vi "example_02_convert.vi"() -> ()   [LabVIEW 2015, in "lv-unit-conversion.lvlib"] (continued)
Kingdom 2240 lbf."}, {"symbol"="tonf[US]", "name"="US ton-force", "dimension"="LM/T2", "is_si_unit"=TRUE, "category"="atom", "base_unit"="N", "conversion_reference"="NIST-SI", "is_exact"=TRUE, "a"=0.0, "b"=8896.443230521, "c"=1.0, "d"=0.0, "underlying_def"="2000 lbf", "description"="2000 lbf"}, {"symbol"="J.m/m2", "name"="joule metre per square metre", "dimension"="LM/T2", "is_si_unit"=TRUE, "category"="derived", "base_unit"="", "conversion_reference"="", "is_exact"=FALSE, "a"=0.0, "b"=0.0, "c"=0.0, "d"=0.0, "underlying_def"="N", "description"=""}, {"symbol"="J/m", "name"="joule per metre", "dimension"="LM/T2", "is_si_unit"=TRUE, "category"="derived", "base_unit"="", "conversion_reference"="", "is_exact"=FALSE, "a"=0.0, "b"=0.0, "c"=0.0, "d"=0.0, "underlying_def"="N", "description"=""}, {"symbol"="N.m/m", "name"="newton metre per metre", "dimension"="LM/T2", "is_si_unit"=TRUE, "category"="derived", "base_unit"="", "conversion_reference"="", "is_exact"=FALSE, "a"=0.0, "b"=0.0, "c"=0.0, "d"=0.0, "underlying_def"="N", "description"=""}, {"symbol"="kcal[th].m/cm2", "name"="thousand calorie metre per square centimetre", "dimension"="LM/T2", "is_si_unit"=TRUE, "category"="derived", "base_unit"="J.m/m2", "conversion_reference"="DERIVED", "is_exact"=TRUE, "a"=0.0, "b"=41840000.0, "c"=1.0, "d"=0.0, "underlying_def"="", "description"=""}, {"symbol"="MJ/m", "name"="megajoule per metre", "dimension"="LM/T2", "is_si_unit"=TRUE, "category"="derived", "base_unit"="J/m", "conversion_reference"="DERIVED", "is_exact"=TRUE, "a"=0.0, "b"=1000000.0, "c"=1.0, "d"=0.0, "underlying_def"="", "description"=""}, {"symbol"="10 kN", "name"="ten kilonewton", "dimension"="LM/T2", "is_si_unit"=TRUE, "category"="derived", "base_unit"="N", "conversion_reference"="DERIVED", "is_exact"=TRUE, "a"=0.0, "b"=10000.0, "c"=1.0, "d"=0.0, "underlying_def"="", "description"=""}, {"symbol"="kgf.m/m", "name"="thousand gram-force metre per metre", "dimension"="LM/T2", "is_si_unit"=TRUE, "category"="derived", "base_unit"="N.m/m", "conversion_reference"="DERIVED", "is_exact"=TRUE, "a"=0.0, "b"=9.80665, "c"=1.0, "d"=0.0, "underlying_def"="", "description"=""}, {"symbol"="lbf.ft/in", "name"="foot pound-force per inch", "dimension"="LM/T2", "is_si_unit"=TRUE, "category"="derived", "base_unit"="N.m/m", "conversion_reference"="DERIVED", "is_exact"=TRUE, "a"=0.0, "b"=53.378659383126, "c"=1.0, "d"=0.0, "underlying_def"="", "description"="Equivalent to \"12 lbf\"."}, {"symbol"="lbf.in/in", "name"="pound-force inch per inch", "dimension"="LM/T2", "is_si_unit"=TRUE, "category"="derived", "base_unit"="N.m/m", "conversion_reference"="DERIVED", "is_exact"=TRUE, "a"=0.0, "b"=4.4482216152605, "c"=1.0, "d"=0.0, "underlying_def"="", "description"=""}, {"symbol"="tonf[US].mi/ft", "name"="US ton-force mile per foot", "dimension"="LM/T2", "is_si_unit"=TRUE, "category"="derived", "base_unit"="N.m/m", "conversion_reference"="DERIVED", "is_exact"=TRUE, "a"=0.0, "b"=46973220.25715088, "c"=1.0, "d"=0.0, "underlying_def"="", "description"="Equivalent to \"5280 tonf[US]\"."}, {"symbol"="cN", "name"="centinewton", "dimension"="LM/T2", "is_si_unit"=TRUE, "category"="prefixed", "base_unit"="N", "conversion_reference"="DERIVED", "is_exact"=TRUE, "a"=0.0, "b"=0.01, "c"=1.0, "d"=0.0, "underlying_def"="", "description"=""}, {"symbol"="daN", "name"="dekanewton", "dimension"="LM/T2", "is_si_unit"=TRUE, "category"="prefixed", "base_unit"="N", "conversion_reference"="DERIVED", "is_exact"=TRUE, "a"=0.0, "b"=10.0, "c"=1.0, "d"=0.0, "underlying_def"="", "description"=""}, {"symbol"="dN", "name"="decinewton", "dimension"="LM/T2", "is_si_unit"=TRUE, "category"="prefixed", "base_unit"="N", "conversion_reference"="DERIVED", "is_exact"=TRUE, "a"=0.0, "b"=0.1, "c"=1.0, "d"=0.0, "underlying_def"="", "description"=""}, {"symbol"="EN", "name"="exanewton", "dimension"="LM/T2", "is_si_unit"=TRUE, "category"="prefixed", "base_unit"="N", "conversion_reference"="DERIVED", "is_exact"=TRUE, "a"=0.0, "b"=1e+18, "c"=1.0, "d"=0.0, "underlying_def"="", "description"=""}, {"symbol"="fN", "name"="femtonewton", "dimension"="LM/T2", "is_si_unit"=TRUE, "category"="prefixed", "base_unit"="N", "conversion_reference"="DERIVED", "is_exact"=TRUE, "a"=0.0, "b"=1e-15, "c"=1.0, "d"=0.0, "underlying_def"="", "description"=""}, {"symbol"="GN", "name"="giganewton", "dimension"="LM/T2", "is_si_unit"=TRUE, "category"="prefixed", "base_unit"="N", "conversion_reference"="DERIVED", "is_exact"=TRUE, "a"=0.0, "b"=1000000000.0, "c"=1.0, "d"=0.0, "underlying_def"="", "description"=""}, {"symbol"="hN", "name"="hectonewton", "dimension"="LM/T2", "is_si_unit"=TRUE, "category"="prefixed", "base_unit"="N", "conversion_reference"="DERIVED", "is_exact"=TRUE, "a"=0.0, "b"=100.0, "c"=1.0, "d"=0.0, "underlying_def"="", "description"=""}, {"symbol"="kdyne", "name"="kilodyne", "dimension"="LM/T2", "is_si_unit"=TRUE, "category"="prefixed", "base_unit"="N", "conversion_reference"="DERIVED", "is_exact"=TRUE, "a"=0.0, "b"=0.01, "c"=1.0, "d"=0.0, "underlying_def"="", "description"=""}, {"symbol"="kgf", "name"="thousand gram-force", "dimension"="LM/T2", "is_si_unit"=TRUE, "category"="prefixed", "base_unit"="N", "conversion_reference"="DERIVED", "is_exact"=TRUE, "a"=0.0, "b"=9.80665, "c"=1.0, "d"=0.0, "underlying_def"="", "description"=""}, {"symbol"="klbf", "name"="thousand pound-force", "dimension"="LM/T2", "is_si_unit"=TRUE, "category"="prefixed", "base_unit"="N", "conversion_reference"="DERIVED", "is_exact"=TRUE, "a"=0.0, "b"=4448.2216152605, "c"=1.0, "d"=0.0, "underlying_def"="", "description"=""}, {"symbol"="kN", "name"="kilonewton", "dimension"="LM/T2", "is_si_unit"=TRUE, "category"="prefixed", "base_unit"="N", "conversion_reference"="DERIVED", "is_exact"=TRUE, "a"=0.0, "b"=1000.0, "c"=1.0, "d"=0.0, "underlying_def"="", "description"=""}, {"symbol"="Mgf", "name"="million gram-force", "dimension"="LM/T2", "is_si_unit"=TRUE, "category"="prefixed", "base_unit"="N", "conversion_reference"="DERIVED", "is_exact"=TRUE, "a"=0.0, "b"=9806.65, "c"=1.0, "d"=0.0, "underlying_def"="", "description"=""}, {"symbol"="mN", "name"="millinewton", "dimension"="LM/T2", "is_si_unit"=TRUE, "category"="prefixed", "base_unit"="N", "conversion_reference"="DERIVED", "is_exact"=TRUE, "a"=0.0, "b"=0.001, "c"=1.0, "d"=0.0, "underlying_def"="", "description"=""}, {"symbol"="MN", "name"="meganewton", "dimension"="LM/T2", "is_si_unit"=TRUE, "category"="prefixed", "base_unit"="N", "conversion_reference"="DERIVED", "is_exact"=TRUE, "a"=0.0, "b"=1000000.0, "c"=1.0, "d"=0.0, "underlying_def"="", "description"=""}, {"symbol"="nN", "name"="nanonewton", "dimension"="LM/T2", "is_si_unit"=TRUE, "category"="prefixed", "base_unit"="N", "conversion_reference"="DERIVED", "is_exact"=TRUE, "a"=0.0, "b"=1e-09, "c"=1.0, "d"=0.0, "underlying_def"="", "description"=""}, {"symbol"="pN", "name"="piconewton", "dimension"="LM/T2", "is_si_unit"=TRUE, "category"="prefixed", "base_unit"="N", "conversion_reference"="DERIVED", "is_exact"=TRUE, "a"=0.0, "b"=1e-12, "c"=1.0, "d"=0.0, "underlying_def"="", "description"=""}, {"symbol"="TN", "name"="teranewton", "dimension"="LM/T2", "is_si_unit"=TRUE, "category"="prefixed", "base_unit"="N", "conversion_reference"="DERIVED", "is_exact"=TRUE, "a"=0.0, "b"=1000000000000.0, "c"=1.0, "d"=0.0, "underlying_def"="", "description"=""}, {"symbol"="uN", "name"="micronewton", "dimension"="LM/T2", "is_si_unit"=TRUE, "category"="prefixed", "base_unit"="N", "conversion_reference"="DERIVED", "is_exact"=TRUE, "a"=0.0, "b"=1e-06, "c"=1.0, "d"=0.0, "underlying_def"="", "description"=""}, {"symbol"="1/bar", "name"="per bar", "dimension"="LT2/M", "is_si_unit"=TRUE, "category"="derived", "base_unit"="1/Pa", "conversion_reference"="DERIVED", "is_exact"=TRUE, "a"=0.0, "b"=1e-05, "c"=1.0, "d"=0.0, "underlying_def"="", "description"=""}, {"symbol"="1/kPa", "name"="per kilopascal", "dimension"="LT2/M", "is_si_unit"=TRUE, "category"="derived", "base_unit"="1/Pa", "conversion_reference"="DERIVED", "is_exact"=TRUE, "a"=0.0, "b"=0.001, "c"=1.0, "d"=0.0, "underlying_def"="", "description"=""}, {"symbol"="1/pPa", "name"="per picopascal", "dimension"="LT2/M", "is_si_unit"=TRUE, "category"="derived", "base_unit"="1/Pa", "conversion_reference"="DERIVED", "is_exact"=TRUE, "a"=0.0, "b"=1000000000000.0, "c"=1.0, "d"=0.0, "underlying_def"="", "description"=""}, {"symbol"="1/psi", "name"="per psi", "dimension"="LT2/M", "is_si_unit"=TRUE, "category"="derived", "base_unit"="1/Pa", "conversion_reference"="DERIVED", "is_exact"=TRUE, "a"=0.0, "b"=0.00064516, "c"=4.4482216152605, "d"=0.0, "underlying_def"="", "description"=""}, {"symbol"="1/upsi", "name"="per millionth of psi", "dimension"="LT2/M", "is_si_unit"=TRUE, "category"="derived", "base_unit"="1/Pa", "conversion_reference"="DERIVED", "is_exact"=TRUE, "a"=0.0, "b"=645.16, "c"=4.4482216152605, "d"=0.0, "underlying_def"="", "description"=""}, {"symbol"="1/Pa", "name"="per pascal", "dimension"="LT2/M", "is_si_unit"=TRUE, "category"="derived", "base_unit"="", "conversion_reference"="", "is_exact"=FALSE, "a"=0.0, "b"=0.0, "c"=0.0, "d"=0.0, "underlying_def"="", "description"=""}, {"symbol"="m3/J", "name"="cubic metre per joule", "dimension"="LT2/M", "is_si_unit"=TRUE, "category"="derived", "base_unit"="", "conversion_reference"="", "is_exact"=FALSE, "a"=0.0, "b"=0.0, "c"=0.0, "d"=0.0, "underlying_def"="1/Pa", "description"=""}, {"symbol"="dm3/(kW.h)", "name"="cubic decimetre per kilowatt hour", "dimension"="LT2/M", "is_si_unit"=TRUE, "category"="derived", "base_unit"="m3/J", "conversion_reference"="DERIVED", "is_exact"=TRUE, "a"=0.0, "b"=0.001, "c"=3600000.0, "d"=0.0, "underlying_def"="", "description"=""}, {"symbol"="dm3/MJ", "name"="cubic decimetre per megajoule", "dimension"="LT2/M", "is_si_unit"=TRUE, "category"="derived", "base_unit"="m3/J", "conversion_reference"="DERIVED", "is_exact"=TRUE, "a"=0.0, "b"=1e-09, "c"=1.0, "d"=0.0, "underlying_def"="", "description"=""}, {"symbol"="m3/(kW.h)", "name"="cubic metre per kilowatt hour", "dimension"="LT2/M", "is_si_unit"=TRUE, "category"="derived", "base_unit"="m3/J", "conversion_reference"="DERIVED", "is_exact"=TRUE, "a"=0.0, "b"=1.0, "c"=3600000.0, "d"=0.0, "underlying_def"="", "description"=""}, {"symbol"="mm3/J", "name"="cubic millimetre per joule", "dimension"="LT2/M", "is_si_unit"=TRUE, "category"="derived", "base_unit"="m3/J", "conversion_reference"="DERIVED", "is_exact"=TRUE, "a"=0.0, "b"=1e-09, "c"=1.0, "d"=0.0, "underlying_def"="", "description"=""}, {"symbol"="pt[UK]/(hp.h)", "name"="UK pint per horsepower hour", "dimension"="LT2/M", "is_si_unit"=TRUE, "category"="derived", "base_unit"="m3/J", "conversion_reference"="DERIVED", "is_exact"=TRUE, "a"=0.0, "b"=0.00056826125, "c"=2684519.537696173, "d"=0.0, "underlying_def"="", "description"=""}, {"symbol"="ct", "name"="carat", "dimension"="M", "is_si_unit"=TRUE, "category"="atom", "base_unit"="kg", "conversion_reference"="NIST-SI", "is_exact"=TRUE, "a"=0.0, "b"=0.0002, "c"=1.0, "d"=0.0, "underlying_def"="200 mg", "description"="200 milligrams (exactly), from NIST-44."}, {"symbol"="cwt[UK]", "name"="UK hundredweight", "dimension"="M", "is_si_unit"=TRUE, "category"="atom", "base_unit"="kg", "conversion_reference"="UK-1995", "is_exact"=TRUE, "a"=0.0, "b"=50.80234544, "c"=1.0, "d"=0.0, "underlying_def"="112 lbm", "description"="United Kingdom 112 pound-mass Gross or long hundredweight. From NIST-44."}, {"symbol"="cwt[US]", "name"="US hundredweight", "dimension"="M", "is_si_unit"=TRUE, "category"="atom", "base_unit"="kg", "conversion_reference"="NIST-44", "is_exact"=TRUE, "a"=0.0, "b"=45.359237, "c"=1.0, "d"=0.0, "underlying_def"="100 lbm", "description"="100 lbm. Net or short hundredweight. From NIST-44."}, {"symbol"="g", "name"="gram", "dimension"="M", "is_si_unit"=TRUE, "category"="atom-base", "base_unit"="kg", "conversion_reference"="NIST-SI", "is_exact"=TRUE, "a"=0.0, "b"=0.001, "c"=1.0, "d"=0.0, "underlying_def"="1/1000 kg", "description"="One thousandth of a kilogram."}, {"symbol"="grain", "name"="grain", "dimension"="M", "is_si_unit"=TRUE, "category"="atom", "base_unit"="kg", "conversion_reference"="NIST-44", "is_exact"=TRUE, "a"=0.0, "b"=6.479891e-05, "c"=1.0, "d"=0.0, "underlying_def"="", "description"="The \"grain\" is the same in avoirdupois, troy, and apothecaries units of mass."}, {"symbol"="lbm", "name"="pound-mass", "dimension"="M", "is_si_unit"=TRUE, "category"="atom", "base_unit"="kg", "conversion_reference"="NIST-SI", "is_exact"=TRUE, "a"=0.0, "b"=0.45359237, "c"=1.0, "d"=0.0, "underlying_def"="", "description"="International avoirdupois pound."}, {"symbol"="ozm", "name"="ounce-mass", "dimension"="M", "is_si_unit"=TRUE, "category"="atom", "base_unit"="kg", "conversion_reference"="NIST-44", "is_exact"=TRUE, "a"=0.0, "b"=0.45359237, "c"=16.0, "d"=0.0, "underlying_def"="1/16 lbm", "description"="One sixteenth of an International avoirdupois pound (lbm)."}, {"symbol"="ozm[troy]", "name"="troy ounce-mass", "dimension"="M", "is_si_unit"=TRUE, "category"="atom", "base_unit"="kg", "conversion_reference"="NIST-44", "is_exact"=TRUE, "a"=0.0, "b"=0.0311034768, "c"=1.0, "d"=0.0, "underlying_def"="480 grain", "description"="Apothecaries or Troy ounce"}, {"symbol"="sack[94lbm]", "name"="94 pound-mass sack", "dimension"="M", "is_si_unit"=TRUE, "category"="atom", "base_unit"="kg", "conversion_reference"="DEFINITION", "is_exact"=TRUE, "a"=0.0, "b"=42.63768278, "c"=1.0, "d"=0.0, "underlying_def"="94 lbm", "description"="A sack with a nominal weight of 94 pound-mass. \n\t\t\t\tWhile the conversion of 94 lbm is exact, the weight of the sack is not exactly 94 lbm.\n\t\t\t"}, {"symbol"="t", "name"="tonne", "dimension"="M", "is_si_unit"=TRUE, "category"="atom-allowed", "base_unit"="kg", "conversion_reference"="NIST-SI", "is_exact"=TRUE, "a"=0.0, "b"=1000.0, "c"=1.0, "d"=0.0, "underlying_def"="1000 kg", "description"="In the US, this is called a metric ton."}, {"symbol"="ton[UK]", "name"="UK ton-mass", "dimension"="M", "is_si_unit"=TRUE, "category"="atom", "base_unit"="kg", "conversion_reference"="NIST-44", "is_exact"=TRUE, "a"=0.0, "b"=1016.0469088, "c"=1.0, "d"=0.0, "underlying_def"="2240 lbm", "description"="Gross or long ton."}, {"symbol"="ton[US]", "name"="US ton-mass", "dimension"="M", "is_si_unit"=TRUE, "category"="atom", "base_unit"="kg", "conversion_reference"="NIST-44", "is_exact"=TRUE, "a"=0.0, "b"=907.18474, "c"=1.0, "d"=0.0, "underlying_def"="2000 lbm", "description"="Net or short ton."}, {"symbol"="kg", "name"="kilogram", "dimension"="M", "is_si_unit"=TRUE, "category"="prefixed", "base_unit"="", "conversion_reference"="", "is_exact"=FALSE, "a"=0.0, "b"=0.0, "c"=0.0, "d"=0.0, "underlying_def"="", "description"="The kilogram is the unit of mass (not force); it is equal to the mass of the international prototype \n\t\t\t\tof the kilogram.\n\t\t\t"}, {"symbol"="ag", "name"="attogram", "dimension"="M", "is_si_unit"=TRUE, "category"="prefixed", "base_unit"="kg", "conversion_reference"="DERIVED", "is_exact"=TRUE, "a"=0.0, "b"=1e-21, "c"=1.0, "d"=0.0, "underlying_def"="", "description"=""}, {"symbol"="cg", "name"="centigram", "dimension"="M", "is_si_unit"=TRUE, "category"="prefixed", "base_unit"="kg", "conversion_reference"="DERIVED", "is_exact"=TRUE, "a"=0.0, "b"=1e-05, "c"=1.0, "d"=0.0, "underlying_def"="", "description"=""}, {"symbol"="Eg", "name"="exagram", "dimension"="M", "is_si_unit"=TRUE, "category"="prefixed", "base_unit"="kg", "conversion_reference"="DERIVED", "is_exact"=TRUE, "a"=0.0, "b"=1000000000000000.0, "c"=1.0, "d"=0.0, "underlying_def"="", "description"=""}, {"symbol"="fg", "name"="femtogram", "dimension"="M", "is_si_unit"=TRUE, "category"="prefixed", "base_unit"="kg", "conversion_reference"="DERIVED", "is_exact"=TRUE, "a"=0.0, "b"=1e-18, "c"=1.0, "d"=0.0, "underlying_def"="", "description"=""}, {"symbol"="Gg", "name"="gigagram", "dimension"="M", "is_si_unit"=TRUE, "category"="prefixed", "base_unit"="kg", "conversion_reference"="DERIVED", "is_exact"=TRUE, "a"=0.0, "b"=1000000.0, "c"=1.0, "d"=0.0, "underlying_def"="", "description"=""}, {"symbol"="hg", "name"="hectogram", "dimension"="M", "is_si_unit"=TRUE, "category"="prefixed", "base_unit"="kg", "conversion_reference"="DERIVED", "is_exact"=TRUE, "a"=0.0, "b"=0.1, "c"=1.0, "d"=0.0, "underlying_def"="", "description"=""}, {"symbol"="klbm", "name"="thousand pound-mass", "dimension"="M", "is_si_unit"=TRUE, "category"="prefixed", "base_unit"="kg", "conversion_reference"="NIST-44", "is_exact"=TRUE, "a"=0.0, "b"=453.59237, "c"=1.0, "d"=0.0, "underlying_def"="", "description"="1000 lbm."}, {"symbol"="mg", "name"="milligram", "dimension"="M", "is_si_unit"=TRUE, "category"="prefixed", "base_unit"="kg", "conversion_reference"="DERIVED", "is_exact"=TRUE, "a"=0.0, "b"=1e-06, "c"=1.0, "d"=0.0, "underlying_def"="", "description"=""}, {"symbol"="Mg", "name"="megagram", "dimension"="M", "is_si_unit"=TRUE, "category"="prefixed", "base_unit"="kg", "conversion_reference"="DERIVED", "is_exact"=TRUE, "a"=0.0, "b"=1000.0, "c"=1.0, "d"=0.0, "underlying_def"="", "description"=""}, {"symbol"="ng", "name"="nanogram", "dimension"="M", "is_si_unit"=TRUE, "category"="prefixed", "base_unit"="kg", "conversion_reference"="DERIVED", "is_exact"=TRUE, "a"=0.0, "b"=1e-12, "c"=1.0, "d"=0.0, "underlying_def"="", "description"=""}, {"symbol"="pg", "name"="picogram", "dimension"="M", "is_si_unit"=TRUE, "category"="prefixed", "base_unit"="kg", "conversion_reference"="DERIVED", "is_exact"=TRUE, "a"=0.0, "b"=1e-15, "c"=1.0, "d"=0.0, "underlying_def"="", "description"=""}, {"symbol"="Tg", "name"="teragram", "dimension"="M", "is_si_unit"=TRUE, "category"="prefixed", "base_unit"="kg", "conversion_reference"="DERIVED", "is_exact"=TRUE, "a"=0.0, "b"=1000000000.0, "c"=1.0, "d"=0.0, "underlying_def"="", "description"=""}, {"symbol"="ug", "name"="microgram", "dimension"="M", "is_si_unit"=TRUE, "category"="prefixed", "base_unit"="kg", "conversion_reference"="DERIVED", "is_exact"=TRUE, "a"=0.0, "b"=1e-09, "c"=1.0, "d"=0.0, "underlying_def"="", "description"=""}, {"symbol"="W/(m3.deltaK)", "name"="watt per cubic metre delta kelvin", "dimension"="M/DLT3", "is_si_unit"=TRUE, "category"="derived", "base_unit"="", "conversion_reference"="", "is_exact"=FALSE, "a"=0.0, "b"=0.0, "c"=0.0, "d"=0.0, "underlying_def"="", "description"=""}, {"symbol"="Btu[IT]/(h.ft3.deltaF)", "name"="BTU per hour cubic foot delta Fahrenheit", "dimension"="M/DLT3", "is_si_unit"=TRUE, "category"="derived", "base_unit"="W/(m3.deltaK)", "conversion_reference"="DERIVED", "is_exact"=TRUE, "a"=0.0, "b"=9495.50267358, "c"=509.703238656, "d"=0.0, "underlying_def"="", "description"=""}, {"symbol"="Btu[IT]/(s.ft3.deltaF)", "name"="(BTU per second) per cubic foot delta Fahrenheit", "dimension"="M/DLT3", "is_si_unit"=TRUE, "category"="derived", "base_unit"="W/(m3.deltaK)", "conversion_reference"="DERIVED", "is_exact"=TRUE, "a"=0.0, "b"=9495.50267358, "c"=0.14158423296, "d"=0.0, "underlying_def"="", "description"=""}, {"symbol"="kW/(m3.deltaK)", "name"="killowatt per cubic metre delta kelvin", "dimension"="M/DLT3", "is_si_unit"=TRUE, "category"="derived", "base_unit"="W/(m3.deltaK)", "conversion_reference"="DERIVED", "is_exact"=TRUE, "a"=0.0, "b"=1000.0, "c"=1.0, "d"=0.0, "underlying_def"="", "description"=""}, {"symbol"="W/(m2.deltaK)", "name"="watt per square metre delta kelvin", "dimension"="M/DT3", "is_si_unit"=TRUE, "category"="derived", "base_unit"="", "conversion_reference"="", "is_exact"=FALSE, "a"=0.0, "b"=0.0, "c"=0.0, "d"=0.0, "underlying_def"="", "description"=""}, {"symbol"="Btu[IT]/(h.ft2.deltaF)", "name"="BTU per hour square foot delta Fahrenheit", "dimension"="M/DT3", "is_si_unit"=TRUE, "category"="derived", "base_unit"="W/(m2.deltaK)", "conversion_reference"="DERIVED", "is_exact"=TRUE, "a"=0.0, "b"=9495.50267358, "c"=1672.25472, "d"=0.0, "underlying_def"="", "description"=""}, {"symbol"="Btu[IT]/(h.ft2.deltaR)", "name"="BTU per hour square foot delta Rankine", "dimension"="M/DT3", "is_si_unit"=TRUE, "category"="derived", "base_unit"="W/(m2.deltaK)", "conversion_reference"="DERIVED", "is_exact"=TRUE, "a"=0.0, "b"=9495.50267358, "c"=1672.25472, "d"=0.0, "underlying_def"="", "description"=""}, {"symbol"="Btu[IT]/(h.m2.deltaC)", "name"="BTU per hour square metre delta Celsius", "dimension"="M/DT3", "is_si_unit"=TRUE, "category"="derived", "base_unit"="W/(m2.deltaK)", "conversion_reference"="DERIVED", "is_exact"=TRUE, "a"=0.0, "b"=1055.05585262, "c"=3600.0, "d"=0.0, "underlying_def"="", "description"=""}, {"symbol"="Btu[IT]/(s.ft2.deltaF)", "name"="(BTU per second) per square foot delta Fahrenheit", "dimension"="M/DT3", "is_si_unit"=TRUE, "category"="derived", "base_unit"="W/(m2.deltaK)", "conversion_reference"="DERIVED", "is_exact"=TRUE, "a"=0.0, "b"=9495.50267358, "c"=0.4645152, "d"=0.0, "underlying_def"="", "description"=""}, {"symbol"="cal[th]/(h.cm2.deltaC)", "name"="calorie per hour square centimetre delta Celsius", "dimension"="M/DT3", "is_si_unit"=TRUE, "category"="derived", "base_unit"="W/(m2.deltaK)", "conversion_reference"="DERIVED", "is_exact"=TRUE, "a"=0.0, "b"=41840.0, "c"=3600.0, "d"=0.0, "underlying_def"="", "description"=""}, {"symbol"="cal[th]/(s.cm2.deltaC)", "name"="calorie per second square centimetre delta Celsius", "dimension"="M/DT3", "is_si_unit"=TRUE, "category"="derived", "base_unit"="W/(m2.deltaK)", "conversion_reference"="DERIVED", "is_exact"=TRUE, "a"=0.0, "b"=41840.0, "c"=1.0, "d"=0.0, "underlying_def"="", "description"=""}, {"symbol"="J/(s.m2.deltaC)", "name"="joule per second square metre delta Celsius", "dimension"="M/DT3", "is_si_unit"=TRUE, "category"="derived", "base_unit"="W/(m2.deltaK)", "conversion_reference"="DERIVED", "is_exact"=TRUE, "a"=0.0, "b"=1.0, "c"=1.0, "d"=0.0, "underlying_def"="", "description"=""}, {"symbol"="kcal[th]/(h.m2.deltaC)", "name"="thousand calorie per hour square metre delta Celsius", "dimension"="M/DT3", "is_si_unit"=TRUE, "category"="derived", "base_unit"="W/(m2.deltaK)", "conversion_reference"="DERIVED", "is_exact"=TRUE, "a"=0.0, "b"=4184.0, "c"=3600.0, "d"=0.0, "underlying_def"="", "description"=""}, {"symbol"="kJ/(h.m2.deltaK)", "name"="kilojoule per hour square metre delta kelvin", "dimension"="M/DT3", "is_si_unit"=TRUE, "category"="derived", "base_unit"="W/(m2.deltaK)", "conversion_reference"="DERIVED", "is_exact"=TRUE, "a"=0.0, "b"=1000.0, "c"=3600.0, "d"=0.0, "underlying_def"="", "description"=""}, {"symbol"="kW/(m2.deltaK)", "name"="kilowatt per square metre delta kelvin", "dimension"="M/DT3", "is_si_unit"=TRUE, "category"="derived", "base_unit"="W/(m2.deltaK)", "conversion_reference"="DERIVED", "is_exact"=TRUE, "a"=0.0, "b"=1000.0, "c"=1.0, "d"=0.0, "underlying_def"="", "description"=""}, {"symbol"="T/m", "name"="tesla per metre", "dimension"="M/ILT2", "is_si_unit"=TRUE, "category"="derived", "base_unit"="", "conversion_reference"="", "is_exact"=FALSE, "a"=0.0, "b"=0.0, "c"=0.0, "d"=0.0, "underlying_def"="", "description"=""}, {"symbol"="gauss/cm", "name"="gauss per centimetre", "dimension"="M/ILT2", "is_si_unit"=TRUE, "category"="derived", "base_unit"="T/m", "conversion_reference"="DERIVED", "is_exact"=TRUE, "a"=0.0, "b"=0.01, "c"=1.0, "d"=0.0, "underlying_def"="", "description"=""}, {"symbol"="mT/dm", "name"="millitesla per decimetre", "dimension"="M/ILT2", "is_si_unit"=TRUE, "category"="derived", "base_unit"="T/m", "conversion_reference"="DERIVED", "is_exact"=TRUE, "a"=0.0, "b"=0.01, "c"=1.0, "d"=0.0, "underlying_def"="", "description"=""}, {"symbol"="T", "name"="tesla", "dimension"="M/IT2", "is_si_unit"=TRUE, "category"="atom-special", "base_unit"="", "conversion_reference"="", "is_exact"=FALSE, "a"=0.0, "b"=0.0, "c"=0.0, "d"=0.0, "underlying_def"="Wb/m2", "description"="The magnetic flux density of 1 Wb/m2. \n\t\t\t\tAlternatively, it is defined as the magnetic flux density that produces on a 1-m length of wire \n\t\t\t\tcarrying a current of 1A, oriented normal to the flux density, a force of 1 N, magnetic flux density \n\t\t\t\tbeing defined as an axial vector quantity such that the force exerted on an element of current is \n\t\t\t\tequal to the vector product of this element and the magnetic flux density.\n\t\t\t"}, {"symbol"="gauss", "name"="gauss", "dimension"="M/IT2", "is_si_unit"=TRUE, "category"="atom", "base_unit"="T", "conversion_reference"="NIST-SI", "is_exact"=TRUE, "a"=0.0, "b"=0.0001, "c"=1.0, "d"=0.0, "underlying_def"="1E-4 T", "description"="This unit is part of the so-called electromagnetic three-dimensional CGS system and cannot strictly \n\t\t\t\tspeaking be compared to the corresponding SI unit, which has four dimensions when only mechanical \n\t\t\t\tand electric quantities are considered.\n\t\t\t"}, {"symbol"="cgauss", "name"="centigauss", "dimension"="M/IT2", "is_si_unit"=TRUE, "category"="prefixed", "base_unit"="T", "conversion_reference"="DERIVED", "is_exact"=TRUE, "a"=0.0, "b"=1e-06, "c"=1.0, "d"=0.0, "underlying_def"="", "description"=""}, {"symbol"="cT", "name"="centitesla", "dimension"="M/IT2", "is_si_unit"=TRUE, "category"="prefixed", "base_unit"="T", "conversion_reference"="DERIVED", "is_exact"=TRUE, "a"=0.0, "b"=0.01, "c"=1.0, "d"=0.0, "underlying_def"="", "description"=""}, {"symbol"="dgauss", "name"="decigauss", "dimension"="M/IT2", "is_si_unit"=TRUE, "category"="prefixed", "base_unit"="T", "conversion_reference"="DERIVED", "is_exact"=TRUE, "a"=0.0, "b"=1e-05, "c"=1.0, "d"=0.0, "underlying_def"="", "description"=""}, {"symbol"="dT", "name"="decitesla", "dimension"="M/IT2", "is_si_unit"=TRUE, "category"="prefixed", "base_unit"="T", "conversion_reference"="DERIVED", "is_exact"=TRUE, "a"=0.0, "b"=0.1, "c"=1.0, "d"=0.0, "underlying_def"="", "description"=""}, {"symbol"="Egauss", "name"="exagauss", "dimension"="M/IT2", "is_si_unit"=TRUE, "category"="prefixed", "base_unit"="T", "conversion_reference"="DERIVED", "is_exact"=TRUE, "a"=0.0, "b"=100000000000000.0, "c"=1.0, "d"=0.0, "underlying_def"="", "description"=""}, {"symbol"="ET", "name"="exatesla", "dimension"="M/IT2", "is_si_unit"=TRUE, "category"="prefixed", "base_unit"="T", "conversion_reference"="DERIVED", "is_exact"=TRUE, "a"=0.0, "b"=1e+18, "c"=1.0, "d"=0.0, "underlying_def"="", "description"=""}, {"symbol"="fgauss", "name"="femtogauss", "dimension"="M/IT2", "is_si_unit"=TRUE, "category"="prefixed", "base_unit"="T", "conversion_reference"="DERIVED", "is_exact"=TRUE, "a"=0.0, "b"=1e-19, "c"=1.0, "d"=0.0, "underlying_def"="", "description"=""}, {"symbol"="fT", "name"="femtotesla", "dimension"="M/IT2", "is_si_unit"=TRUE, "category"="prefixed", "base_unit"="T", "conversion_reference"="DERIVED", "is_exact"=TRUE, "a"=0.0, "b"=1e-15, "c"=1.0, "d"=0.0, "underlying_def"="", "description"=""}, {"symbol"="Ggauss", "name"="gigagauss", "dimension"="M/IT2", "is_si_unit"=TRUE, "category"="prefixed", "base_unit"="T", "conversion_reference"="DERIVED", "is_exact"=TRUE, "a"=0.0, "b"=100000.0, "c"=1.0, "d"=0.0, "underlying_def"="", "description"=""}, {"symbol"="GT", "name"="gigatesla", "dimension"="M/IT2", "is_si_unit"=TRUE, "category"="prefixed", "base_unit"="T", "conversion_reference"="DERIVED", "is_exact"=TRUE, "a"=0.0, "b"=1000000000.0, "c"=1.0, "d"=0.0, "underlying_def"="", "description"=""}, {"symbol"="kgauss", "name"="kilogauss", "dimension"="M/IT2", "is_si_unit"=TRUE, "category"="prefixed", "base_unit"="T", "conversion_reference"="DERIVED", "is_exact"=TRUE, "a"=0.0, "b"=0.1, "c"=1.0, "d"=0.0, "underlying_def"="", "description"=""}, {"symbol"="kT", "name"="kilotesla", "dimension"="M/IT2", "is_si_unit"=TRUE, "category"="prefixed", "base_unit"="T", "conversion_reference"="DERIVED", "is_exact"=TRUE, "a"=0.0, "b"=1000.0, "c"=1.0, "d"=0.0, "underlying_def"="", "description"=""}, {"symbol"="mgauss", "name"="milligauss", "dimension"="M/IT2", "is_si_unit"=TRUE, "category"="prefixed", "base_unit"="T", "conversion_reference"="DERIVED", "is_exact"=TRUE, "a"=0.0, "b"=1e-07, "c"=1.0, "d"=0.0, "underlying_def"="", "description"=""}, {"symbol"="Mgauss", "name"="megagauss", "dimension"="M/IT2", "is_si_unit"=TRUE, "category"="prefixed", "base_unit"="T", "conversion_reference"="DERIVED", "is_exact"=TRUE, "a"=0.0, "b"=100.0, "c"=1.0, "d"=0.0, "underlying_def"="", "description"=""}, {"symbol"="mT", "name"="millitesla", "dimension"="M/IT2", "is_si_unit"=TRUE, "category"="prefixed", "base_unit"="T", "conversion_reference"="DERIVED", "is_exact"=TRUE, "a"=0.0, "b"=0.001, "c"=1.0, "d"=0.0, "underlying_def"="", "description"=""}, {"symbol"="ngauss", "name"="nanogauss", "dimension"="M/IT2", "is_si_unit"=TRUE, "category"="prefixed", "base_unit"="T", "conversion_reference"="DERIVED", "is_exact"=TRUE, "a"=0.0, "b"=1e-13, "c"=1.0, "d"=0.0, "underlying_def"="", "description"=""}, {"symbol"="nT", "name"="nanotesla", "dimension"="M/IT2", "is_si_unit"=TRUE, "category"="prefixed", "base_unit"="T", "conversion_reference"="DERIVED", "is_exact"=TRUE, "a"=0.0, "b"=1e-09, "c"=1.0, "d"=0.0, "underlying_def"="", "description"=""}, {"symbol"="pgauss", "name"="picogauss", "dimension"="M/IT2", "is_si_unit"=TRUE, "category"="prefixed", "base_unit"="T", "conversion_reference"="DERIVED", "is_exact"=TRUE, "a"=0.0, "b"=1e-16, "c"=1.0, "d"=0.0, "underlying_def"="", "description"=""}, {"symbol"="pT", "name"="picotesla", "dimension"="M/IT2", "is_si_unit"=TRUE, "category"="prefixed", "base_unit"="T", "conversion_reference"="DERIVED", "is_exact"=TRUE, "a"=0.0, "b"=1e-12, "c"=1.0, "d"=0.0, "underlying_def"="", "description"=""}, {"symbol"="Tgauss", "name"="teragauss", "dimension"="M/IT2", "is_si_unit"=TRUE, "category"="prefixed", "base_unit"="T", "conversion_reference"="DERIVED", "is_exact"=TRUE, "a"=0.0, "b"=100000000.0, "c"=1.0, "d"=0.0, "underlying_def"="", "description"=""}, {"symbol"="TT", "name"="teratesla", "dimension"="M/IT2", "is_si_unit"=TRUE, "category"="prefixed", "base_unit"="T", "conversion_reference"="DERIVED", "is_exact"=TRUE, "a"=0.0, "b"=1000000000000.0, "c"=1.0, "d"=0.0, "underlying_def"="", "description"=""}, {"symbol"="ugauss", "name"="microgauss", "dimension"="M/IT2", "is_si_unit"=TRUE, "category"="prefixed", "base_unit"="T", "conversion_reference"="DERIVED", "is_exact"=TRUE, "a"=0.0, "b"=1e-10, "c"=1.0, "d"=0.0, "underlying_def"="", "description"=""}, {"symbol"="uT", "name"="microtesla", "dimension"="M/IT2", "is_si_unit"=TRUE, "category"="prefixed", "base_unit"="T", "conversion_reference"="DERIVED", "is_exact"=TRUE, "a"=0.0, "b"=1e-06, "c"=1.0, "d"=0.0, "underlying_def"="", "description"=""}, {"symbol"="kg/m", "name"="kilogram per metre", "dimension"="M/L", "is_si_unit"=TRUE, "category"="derived", "base_unit"="", "conversion_reference"="", "is_exact"=FALSE, "a"=0.0, "b"=0.0, "c"=0.0, "d"=0.0, "underlying_def"="", "description"=""}, {"symbol"="kg.m/cm2", "name"="kilogram metre per square centimetre", "dimension"="M/L", "is_si_unit"=TRUE, "category"="derived", "base_unit"="kg/m", "conversion_reference"="DERIVED", "is_exact"=TRUE, "a"=0.0, "b"=10000.0, "c"=1.0, "d"=0.0, "underlying_def"="", "description"=""}, {"symbol"="klbm/in", "name"="thousand pound-mass per inch", "dimension"="M/L", "is_si_unit"=TRUE, "category"="derived", "base_unit"="kg/m", "conversion_reference"="DERIVED", "is_exact"=TRUE, "a"=0.0, "b"=453.59237, "c"=0.0254, "d"=0.0, "underlying_def"="", "description"=""}, {"symbol"="lbm/ft", "name"="pound-mass per foot", "dimension"="M/L", "is_si_unit"=TRUE, "category"="derived", "base_unit"="kg/m", "conversion_reference"="DERIVED", "is_exact"=TRUE, "a"=0.0, "b"=0.45359237, "c"=0.3048, "d"=0.0, "underlying_def"="", "description"=""}, {"symbol"="Mg/in", "name"="megagram per inch", "dimension"="M/L", "is_si_unit"=TRUE, "category"="derived", "base_unit"="kg/m", "conversion_reference"="DERIVED", "is_exact"=TRUE, "a"=0.0, "b"=1000.0, "c"=0.0254, "d"=0.0, "underlying_def"="", "description"=""}, {"symbol"="kg/m2", "name"="kilogram per square metre", "dimension"="M/L2", "is_si_unit"=TRUE, "category"="derived", "base_unit"="", "conversion_reference"="", "is_exact"=FALSE, "a"=0.0, "b"=0.0, "c"=0.0, "d"=0.0, "underlying_def"="", "description"=""}, {"symbol"="0.01 lbm/ft2", "name"="pound-mass per hundred square foot", "dimension"="M/L2", "is_si_unit"=TRUE, "category"="derived", "base_unit"="kg/m2", "conversion_reference"="DERIVED", "is_exact"=TRUE, "a"=0.0, "b"=0.45359237, "c"=9.290304, "d"=0.0, "underlying_def"="", "description"=""}, {"symbol"="lbm/ft2", "name"="pound-mass per square foot", "dimension"="M/L2", "is_si_unit"=TRUE, "category"="derived", "base_unit"="kg/m2", "conversion_reference"="DERIVED", "is_exact"=TRUE, "a"=0.0, "b"=0.45359237, "c"=0.09290304, "d"=0.0, "underlying_def"="", "description"=""}, {"symbol"="Mg/m2", "name"="megagram per square metre", "dimension"="M/L2", "is_si_unit"=TRUE, "category"="derived", "base_unit"="kg/m2", "conversion_reference"="DERIVED", "is_exact"=TRUE, "a"=0.0, "b"=1000.0, "c"=1.0, "d"=0.0, "underlying_def"="", "description"=""}, {"symbol"="ton[US]/ft2", "name"="US ton-mass per square foot", "dimension"="M/L2", "is_si_unit"=TRUE, "category"="derived", "base_unit"="kg/m2", "conversion_reference"="DERIVED", "is_exact"=TRUE, "a"=0.0, "b"=907.18474, "c"=0.09290304, "d"=0.0, "underlying_def"="", "description"=""}, {"symbol"="kg/(m2.s)", "name"="kilogram per square metre second", "dimension"="M/L2T", "is_si_unit"=TRUE, "category"="derived", "base_unit"="", "conversion_reference"="", "is_exact"=FALSE, "a"=0.0, "b"=0.0, "c"=0.0, "d"=0.0, "underlying_def"="", "description"=""}, {"symbol"="g.ft/(cm3.s)", "name"="gram foot per cubic centimetre second", "dimension"="M/L2T", "is_si_unit"=TRUE, "category"="derived", "base_unit"="kg/(m2.s)", "conversion_reference"="DERIVED", "is_exact"=TRUE, "a"=0.0, "b"=304.8, "c"=1.0, "d"=0.0, "underlying_def"="", "description"=""}, {"symbol"="g.m/(cm3.s)", "name"="gram metre per cubic centimetre second", "dimension"="M/L2T", "is_si_unit"=TRUE, "category"="derived", "base_unit"="kg/(m2.s)", "conversion_reference"="DERIVED", "is_exact"=TRUE, "a"=0.0, "b"=1000.0, "c"=1.0, "d"=0.0, "underlying_def"="", "description"=""}, {"symbol"="kPa.s/m", "name"="kilopascal second per metre", "dimension"="M/L2T", "is_si_unit"=TRUE, "category"="derived", "base_unit"="kg/(m2.s)", "conversion_reference"="DERIVED", "is_exact"=TRUE, "a"=0.0, "b"=1000.0, "c"=1.0, "d"=0.0, "underlying_def"="", "description"=""}, {"symbol"="lbm/(ft2.h)", "name"="pound-mass per square foot hour", "dimension"="M/L2T", "is_si_unit"=TRUE, "category"="derived", "base_unit"="kg/(m2.s)", "conversion_reference"="DERIVED", "is_exact"=TRUE, "a"=0.0, "b"=0.45359237, "c"=334.450944, "d"=0.0, "underlying_def"="", "description"=""}, {"symbol"="lbm/(ft2.s)", "name"="pound-mass per square foot second", "dimension"="M/L2T", "is_si_unit"=TRUE, "category"="derived", "base_unit"="kg/(m2.s)", "conversion_reference"="DERIVED", "is_exact"=TRUE, "a"=0.0, "b"=0.45359237, "c"=0.09290304, "d"=0.0, "underlying_def"="", "description"=""}, {"symbol"="MPa.s/m", "name"="megapascal second per metre", "dimension"="M/L2T", "is_si_unit"=TRUE, "category"="derived", "base_unit"="kg/(m2.s)", "conversion_reference"="DERIVED", "is_exact"=TRUE, "a"=0.0, "b"=1000000.0, "c"=1.0, "d"=0.0, "underlying_def"="", "description"=""}, {"symbol"="N/m3", "name"="newton per cubic metre", "dimension"="M/L2T2", "is_si_unit"=TRUE, "category"="derived", "base_unit"="", "conversion_reference"="", "is_exact"=FALSE, "a"=0.0, "b"=0.0, "c"=0.0, "d"=0.0, "underlying_def"="", "description"=""}, {"symbol"="0.001 psi/ft", "name"="psi per thousand foot", "dimension"="M/L2T2", "is_si_unit"=TRUE, "category"="derived", "base_unit"="N/m3", "conversion_reference"="DERIVED", "is_exact"=TRUE, "a"=0.0, "b"=4.4482216152605, "c"=0.196644768, "d"=0.0, "underlying_def"="", "description"=""}, {"symbol"="0.01 psi/ft", "name"="psi per hundred foot", "dimension"="M/L2T2", "is_si_unit"=TRUE, "category"="derived", "base_unit"="N/m3", "conversion_reference"="DERIVED", "is_exact"=TRUE, "a"=0.0, "b"=4.4482216152605, "c"=0.0196644768, "d"=0.0, "underlying_def"="", "description"=""}, {"symbol"="atm/ft", "name"="standard atmosphere per foot", "dimension"="M/L2T2", "is_si_unit"=TRUE, "category"="derived", "base_unit"="N/m3", "conversion_reference"="DERIVED", "is_exact"=TRUE, "a"=0.0, "b"=101325.0, "c"=0.3048, "d"=0.0, "underlying_def"="", "description"=""}, {"symbol"="atm/hm", "name"="standard atmosphere per hundred metre", "dimension"="M/L2T2", "is_si_unit"=TRUE, "category"="derived", "base_unit"="N/m3", "conversion_reference"="DERIVED", "is_exact"=TRUE, "a"=0.0, "b"=1013.25, "c"=1.0, "d"=0.0, "underlying_def"="", "description"=""}, {"symbol"="atm/m", "name"="standard atmosphere per metre", "dimension"="M/L2T2", "is_si_unit"=TRUE, "category"="derived", "base_unit"="N/m3", "conversion_reference"="DERIVED", "is_exact"=TRUE, "a"=0.0, "b"=101325.0, "c"=1.0, "d"=0.0, "underlying_def"="", "description"=""}, {"symbol"="bar/km", "name"="bar per kilometre", "dimension"="M/L2T2", "is_si_unit"=TRUE, "category"="derived", "base_unit"="N/m3", "conversion_reference"="DERIVED", "is_exact"=TRUE, "a"=0.0, "b"=100.0, "c"=1.0, "d"=0.0, "underlying_def"="", "description"=""}, {"symbol"="bar/m", "name"="bar per metre", "dimension"="M/L2T2", "is_si_unit"=TRUE, "category"="derived", "base_unit"="N/m3", "conversion_reference"="DERIVED", "is_exact"=TRUE, "a"=0.0, "b"=100000.0, "c"=1.0, "d"=0.0, "underlying_def"="", "description"=""}, {"symbol"="GPa/cm", "name"="gigapascal per centimetre", "dimension"="M/L2T2", "is_si_unit"=TRUE, "category"="derived", "base_unit"="N/m3", "conversion_reference"="DERIVED", "is_exact"=TRUE, "a"=0.0, "b"=100000000000.0, "c"=1.0, "d"=0.0, "underlying_def"="", "description"=""}, {"symbol"="kPa/hm", "name"="kilopascal per hectometre", "dimension"="M/L2T2", "is_si_unit"=TRUE, "category"="derived", "base_unit"="N/m3", "conversion_reference"="DERIVED", "is_exact"=TRUE, "a"=0.0, "b"=10.0, "c"=1.0, "d"=0.0, "underlying_def"="", "description"=""}, {"symbol"="kPa/m", "name"="kilopascal per metre", "dimension"="M/L2T2", "is_si_unit"=TRUE, "category"="derived", "base_unit"="N/m3", "conversion_reference"="DERIVED", "is_exact"=TRUE, "a"=0.0, "b"=1000.0, "c"=1.0, "d"=0.0, "underlying_def"="", "description"=""}, {"symbol"="lbf/ft3", "name"="pound-force per cubic foot", "dimension"="M/L2T2", "is_si_unit"=TRUE, "category"="derived", "base_unit"="N/m3", "conversion_reference"="DERIVED", "is_exact"=TRUE, "a"=0.0, "b"=4.4482216152605, "c"=0.028316846592, "d"=0.0, "underlying_def"="", "description"=""}, {"symbol"="lbf/gal[US]", "name"="pound-force per US gallon", "dimension"="M/L2T2", "is_si_unit"=TRUE, "category"="derived", "base_unit"="N/m3", "conversion_reference"="DERIVED", "is_exact"=TRUE, "a"=0.0, "b"=4.4482216152605, "c"=0.003785411784, "d"=0.0, "underlying_def"="", "description"=""}, {"symbol"="MPa/m", "name"="megapascal per metre", "dimension"="M/L2T2", "is_si_unit"=TRUE, "category"="derived", "base_unit"="N/m3", "conversion_reference"="DERIVED", "is_exact"=TRUE, "a"=0.0, "b"=1000000.0, "c"=1.0, "d"=0.0, "underlying_def"="", "description"=""}, {"symbol"="Pa/m", "name"="pascal per metre", "dimension"="M/L2T2", "is_si_unit"=TRUE, "category"="derived", "base_unit"="N/m3", "conversion_reference"="DERIVED", "is_exact"=TRUE, "a"=0.0, "b"=1.0, "c"=1.0, "d"=0.0, "underlying_def"="", "description"=""}, {"symbol"="psi/ft", "name"="psi per foot", "dimension"="M/L2T2", "is_si_unit"=TRUE, "category"="derived", "base_unit"="N/m3", "conversion_reference"="DERIVED", "is_exact"=TRUE, "a"=0.0, "b"=4.4482216152605, "c"=0.000196644768, "d"=0.0, "underlying_def"="", "description"=""}, {"symbol"="psi/m", "name"="psi per metre", "dimension"="M/L2T2", "is_si_unit"=TRUE, "category"="derived", "base_unit"="N/m3", "conversion_reference"="DERIVED", "is_exact"=TRUE, "a"=0.0, "b"=4.4482216152605, "c"=0.00064516, "d"=0.0, "underlying_def"="", "description"=""}, {"symbol"="kg/m3", "name"="kilogram per cubic metre", "dimension"="M/L3", "is_si_unit"=TRUE, "category"="derived", "base_unit"="", "conversion_reference"="", "is_exact"=FALSE, "a"=0.0, "b"=0.0, "c"=0.0, "d"=0.0, "underlying_def"="", "description"=""}, {"symbol"="0.001 lbm/bbl", "name"="pound-mass per thousand barrel"
